vi "MI.Get Stage 1 Temperature.vi"(8 "error in (no error)":errorcluster, 11 "TCP Network Connection in":refnum<k5>) -> (0 "error out":errorcluster, 2 "Stage 1 Temperature (K)":dbl, 3 "TCP Network Connection out":refnum<k5>)   [LabVIEW 2016, in "instrument.Cryostation.lvclass"]
uses:
  instrument.Cryostation.lvclass
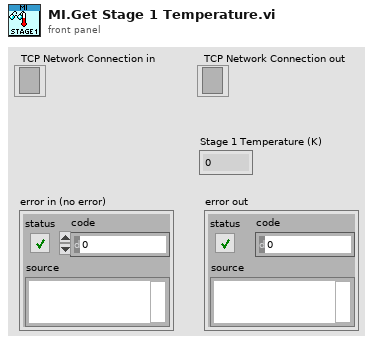
[diagram p1: front panel]
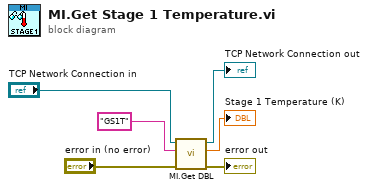
[diagram p0: block diagram]
diagram:
  n1 = call "MI.Get DBL.vi"("error in (no error)"="error in (no error)", "String"="GS1T", "connection ID in"="TCP Network Connection in") -> ("error out"=→"error out":errorcluster, "Numeric"=→"Stage 1 Temperature (K)":dbl, "connection ID out"=→"TCP Network Connection out":refnum<k5>)  [unwired: 6 in]
